vi "N01_While_Loop.vi"() -> ()   [LabVIEW 2023]
panel:
  out "Meter":dbl(knob) scale=0.0..10.0
  out "Boolean 2":bool
  in  "Boolean":bool
  out "Numeric 2":dbl
  in  "Numeric":dbl
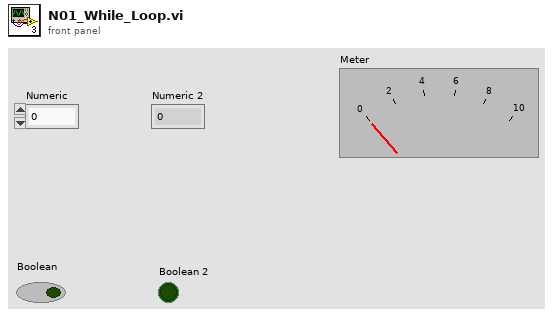
[diagram p1: front panel]
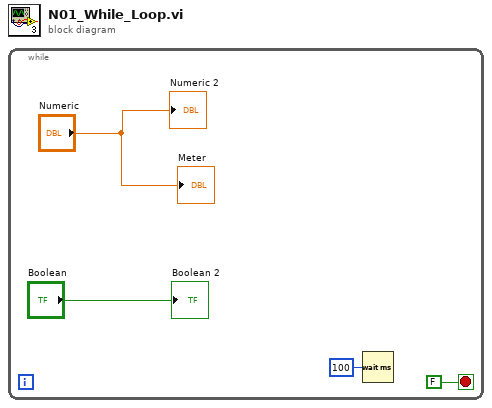
[diagram p0: block diagram]
diagram:
  n1 = while {
    stop <- FALSE stop-if-true
    n2 = Wait (ms)(milliseconds to wait=u32 100) -> ()  [unwired: 1 out]
    "Numeric 2" <- "Numeric"
    "Boolean 2" <- "Boolean"
    "Meter" <- "Numeric"
  }
